vi "5492_WPI_JoystickArcadeMapping.vi"(6 "Max Output":dbl=1.0, 7 "Square Inputs":bool=TRUE, 9 "Y axis value":dbl, 10 "X axis value":dbl, 11 "Orientation Toggle":bool) -> (1 "Right Motor Value":dbl, 2 "Left Motor Value":dbl)   [LabVIEW 2016]
doc: "Uses a standard algorithm to map joystick axes into motor updates for arcade driving. This algorithm does not saturate over half of the range.\n\nThis software is licensed. Open the labview\\readme\\WPI Robotics Library Open Source License.txt file for more information."
uses:
  5492_OrientationButtonPress.vi
  5492_DriveOrientation.vi
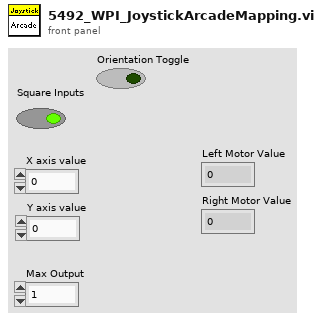
[diagram p1: front panel]
types:
  T1 = typedef "WPI_PWMDeviceRef.ctl" = cluster{"DeviceStatus":errorcluster, "PWM Channel":T2}
  T2 = typedef "FPGA_DIOPWMChannel.ctl" = enum8{"PWM 0", "PWM 1", "PWM 2", "PWM 3", "PWM 4", "PWM 5", "PWM 6", "PWM 7", "PWM 8", "PWM 9", "PWM MXP 0", "PWM MXP 1", "PWM MXP 2", "PWM MXP 3", "PWM MXP 4", "PWM MXP 5", "PWM MXP 6", "PWM MXP 7", "PWM MXP 8", "PWM MXP 9", "Invalid"}
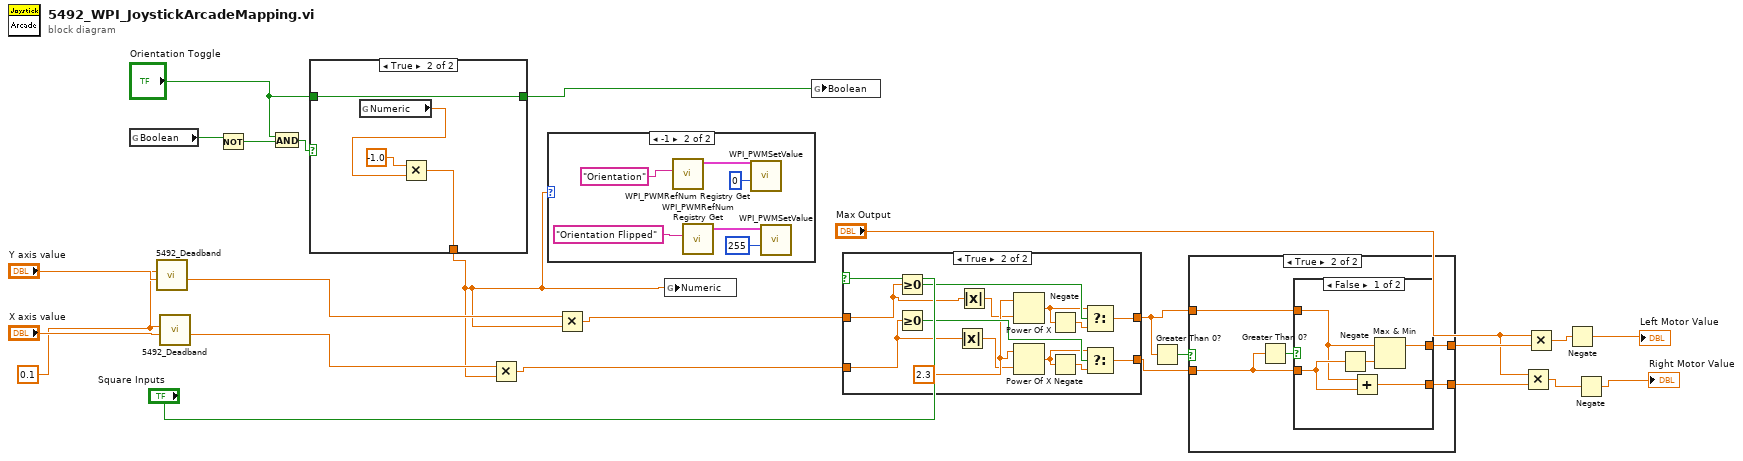
[diagram p0: block diagram]
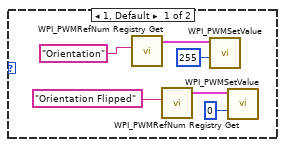
[diagram p2: hidden frame]
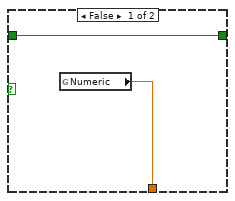
[diagram p3: hidden frame]
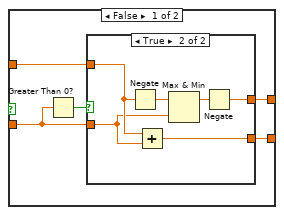
[diagram p4: hidden frame]
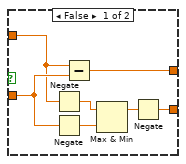
[diagram p5: hidden frame]
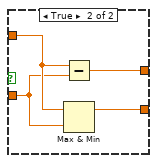
[diagram p6: hidden frame]
diagram:
  w15 = 0.1
  n1 = global read "5492_OrientationButtonPress.vi" "Boolean"() -> (w6:bool)
  n2 = call "5492_Deadband.vi"("Input"="Y axis value", "DeadBand"=w15) -> ("Output"=w10:dbl)  [unwired: 9 in]
  n3 = call "5492_Deadband.vi"("Input"="X axis value", "DeadBand"=w15) -> ("Output"=w9:dbl)  [unwired: 9 in]
  n4 = Not(x=w6) -> (.not. x?=w3:bool)
  n5 = And(x="Orientation Toggle", y=w3) -> (x .and. y?=w5:bool)
  n6 = case shown="True" w5 {
    tunnel: [w26 w28] -> w1
    tunnel: "Orientation Toggle" -> [w25 w27]
    tunnel: [w25 w27] -> w4
    frame False {
      n7 = global read "5492_DriveOrientation.vi" "Numeric"() -> (w26:dbl)
    }
    frame True {
      n8 = global read "5492_DriveOrientation.vi" "Numeric"() -> (w29:dbl)
      n9 = Multiply(x=-1.0, y=w29) -> (x*y=w28:dbl)
    }
  }
  n10 = Multiply(x=w9, y=w1) -> (x*y=w8:dbl)
  n11 = case shown="-1" w1 {
    frame 1, Default {
      n12 = call <vilib>:"WPI_PWMRefNum Registry Get.vi"("refnum name"="Orientation") -> ("PWMDeviceRef"=w36:T1)  [unwired: 9 in, 1 out]
      n13 = call <vilib>:"WPI_PWMRefNum Registry Get.vi"("refnum name"="Orientation Flipped") -> ("PWMDeviceRef"=w35:T1)  [unwired: 9 in, 1 out]
      n14 = call <vilib>:"WPI_PWMSetValue.vi"("Value"=u16 255, "PWMDeviceRef"=w36) -> ()  [unwired: 8 in, 2 out]
      n15 = call <vilib>:"WPI_PWMSetValue.vi"("Value"=u16 0, "PWMDeviceRef"=w35) -> ()  [unwired: 8 in, 2 out]
    }
    frame -1 {
      n16 = call <vilib>:"WPI_PWMRefNum Registry Get.vi"("refnum name"="Orientation") -> ("PWMDeviceRef"=w37:T1)  [unwired: 9 in, 1 out]
      n17 = call <vilib>:"WPI_PWMRefNum Registry Get.vi"("refnum name"="Orientation Flipped") -> ("PWMDeviceRef"=w42:T1)  [unwired: 9 in, 1 out]
      n18 = call <vilib>:"WPI_PWMSetValue.vi"("Value"=u16 0, "PWMDeviceRef"=w37) -> ()  [unwired: 8 in, 2 out]
      n19 = call <vilib>:"WPI_PWMSetValue.vi"("Value"=u16 255, "PWMDeviceRef"=w42) -> ()  [unwired: 8 in, 2 out]
    }
  }
  n20 = Multiply(x=w10, y=w1) -> (x*y=w7:dbl)
  n21 = global write "5492_DriveOrientation.vi" "Numeric"(w1) -> ()
  n22 = global write "5492_OrientationButtonPress.vi" "Boolean"(w4) -> ()
  n23 = case shown="True" "Square Inputs" {
    tunnel: [w43 w57] -> w22
    tunnel: [w44 w56] -> w23
    tunnel: w8 -> [w43 w47]
    tunnel: w7 -> [w44 w45]
    frame False {
    }
    frame True {
      w49 = 2.3
      n24 = Greater Or Equal To 0?(x=w45) -> (x >= 0?=w52:bool)
      n25 = Greater Or Equal To 0?(x=w47) -> (x >= 0?=w55:bool)
      n26 = Absolute Value(x=w47) -> (abs(x)=w48:dbl)
      n27 = Absolute Value(x=w45) -> (abs(x)=w46:dbl)
      n28 = Power Of X(1:w46, 2:w49) -> (0:w50:dbl)
      n29 = Power Of X(1:w48, 2:w49) -> (0:w51:dbl)
      n30 = Negate(x=w50) -> (-x=w53:dbl)
      n31 = Negate(x=w51) -> (-x=w54:dbl)
      n32 = Select(t=w50, s=w52, f=w53) -> (s? t:f=w56:dbl)
      n33 = Select(t=w51, s=w55, f=w54) -> (s? t:f=w57:dbl)
    }
  }
  n34 = Greater Than 0?(x=w23) -> (x > 0?=w24:bool)
  n35 = case shown="True" w24 {
    tunnel: w22 -> [w61 w79]
    tunnel: w23 -> [w60 w78]
    tunnel: [w59 w77] -> w21
    tunnel: [w58 w76] -> w20
    frame False {
      n36 = Greater Than 0?(x=w61) -> (x > 0?=w62:bool)
      n37 = case shown="True" w62 {
        tunnel: w61 -> [w69 w71]
        tunnel: w60 -> [w67 w72]
        tunnel: [w63 w73] -> w59
        tunnel: [w64 w70] -> w58
        frame False {
          n38 = Negate(x=w67) -> (-x=w68:dbl)
          n39 = Negate(x=w69) -> (-x=w66:dbl)
          n40 = Subtract(x=w67, y=w69) -> (x-y=w63:dbl)
          n41 = Max & Min(x=w68, y=w66) -> (max(x,y)=w65:dbl)  [unwired: 1 out]
          n42 = Negate(x=w65) -> (-x=w64:dbl)
        }
        frame True {
          n43 = Negate(x=w72) -> (-x=w75:dbl)
          n44 = Add(x=w72, y=w71) -> (x+y=w70:dbl)
          n45 = Max & Min(x=w75, y=w71) -> (max(x,y)=w74:dbl)  [unwired: 1 out]
          n46 = Negate(x=w74) -> (-x=w73:dbl)
        }
      }
    }
    frame True {
      n47 = Greater Than 0?(x=w79) -> (x > 0?=w80:bool)
      n48 = case shown="False" w80 {
        tunnel: w79 -> [w85 w87]
        tunnel: w78 -> [w82 w88]
        tunnel: [w83 w86] -> w77
        tunnel: [w81 w89] -> w76
        frame False {
          n49 = Negate(x=w85) -> (-x=w84:dbl)
          n50 = Add(x=w82, y=w85) -> (x+y=w81:dbl)
          n51 = Max & Min(x=w82, y=w84) -> (max(x,y)=w83:dbl)  [unwired: 1 out]
        }
        frame True {
          n52 = Subtract(x=w88, y=w87) -> (x-y=w86:dbl)
          n53 = Max & Min(x=w88, y=w87) -> (max(x,y)=w89:dbl)  [unwired: 1 out]
        }
      }
    }
  }
  n54 = Multiply(x="Max Output", y=w20) -> (x*y=w14:dbl)
  n55 = Multiply(x="Max Output", y=w21) -> (x*y=w11:dbl)
  n56 = Negate(x=w11) -> (-x=→"Left Motor Value":dbl)
  n57 = Negate(x=w14) -> (-x=→"Right Motor Value":dbl)
